vi "MK_Steps to Bytes.vi"(11 "Steps":dbl=100.0) -> (2 "Hi Byte":string, 3 "Lo Byte":string)   [LabVIEW 2014]
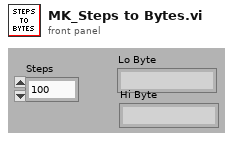
[diagram p1: front panel]
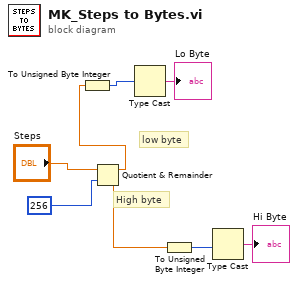
[diagram p0: block diagram]
diagram:
  # "High byte"
  # "low byte"
  n1 = Quotient & Remainder(x="Steps", y=256) -> (x-y*floor(x/y)=w6:dbl, floor(x/y)=w7:dbl)
  n2 = To Unsigned Byte Integer(number=w6) -> (unsigned 8bit integer=w4:u8)
  n3 = Type Cast(x=w4) -> (*(type *) &x=→"Lo Byte":string)  [unwired: 1 in]
  n4 = To Unsigned Byte Integer(number=w7) -> (unsigned 8bit integer=w2:u8)
  n5 = Type Cast(x=w2) -> (*(type *) &x=→"Hi Byte":string)  [unwired: 1 in]
